vi "GetWaveformParentAssetId.vi"(11 "waveform in":waveform(sgl)) -> (1 "found":bool, 2 "parent asset id":string, 3 "waveform out":waveform(sgl))   [LabVIEW 2017]
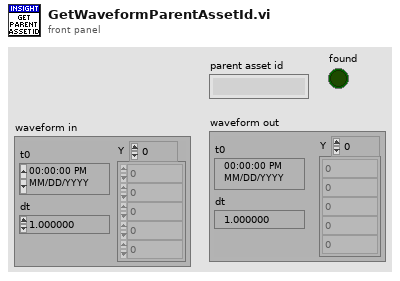
[diagram p1: front panel]
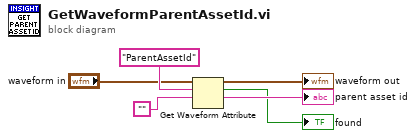
[diagram p0: block diagram]
diagram:
  n1 = Get Waveform Attribute(5:"", 6:"ParentAssetId" ("name"), 7:"waveform in") -> (1:→"parent asset id":string, 2:→"found":bool, 3:→"waveform out":waveform(sgl))  [unwired: 1 in, 1 out]
